vi "Template_Read Index Set.vi"(9 "Default":T1[](array[typedef]), 11 "Indices":i32[](array[numeric])) -> (1 "Values":T1[](array[typedef]))   [LabVIEW 2010, in "Current Value Table.lvlib"]
doc: "This VI reads a set of data as defined by the GetIndices function. This VI can provide an order of magnitude increase in performance over a normal index read for sufficiently large data sets."
uses:
  Template_Datatype.ctl
  Type Defs/Memory Commands.ctl
  I32_Memory Block.vi
  Current Value Table.lvlib
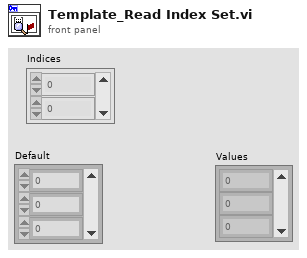
[diagram p1: front panel]
types:
  T1 = typedef "Template_Datatype.ctl" = i32
  T2 = typedef "Current Value Table.lvlib/Memory Commands.ctl" = enum16{"Init", "Add Data", "Read", "Read Group", "Read All", "Write", "Write Group", "Get Size"}
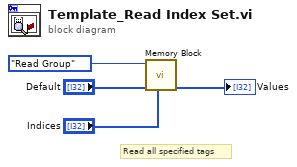
[diagram p0: block diagram]
diagram:
  # "Read all specified tags"
  n1 = call-poly "Memory Block.vi"("Group Indices"="Indices", "Data In"="Default", "Method"=Memory_Commands."Read Group") -> ("Group Data"=→"Values":i32[])  [unwired: 6 in, 2 out]
